vi "Three_Tote.vi"(11 "3_Tote_Enable":bool=TRUE) -> ()   [LabVIEW 2014]
uses:
  General_VI/Global Var.vi
panel:
  in  "Time _To_Drive_1_Tote":i32=8000
  in  "Extend_Flipper_Time":i32=500
  in  "Open_Infeed_time":i32=800
  # "Static Tunning Values"
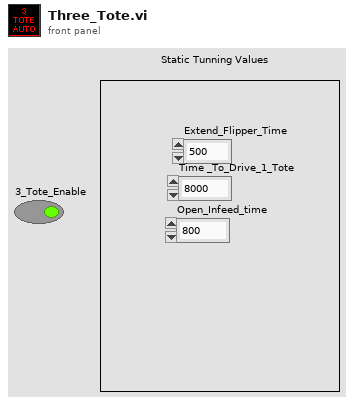
[diagram p1: front panel]
types:
  T1 = cluster{"Open_Infeed_time":i32, "Extend_Flipper_Time":i32, "Time _To_Drive_1_Tote":i32}
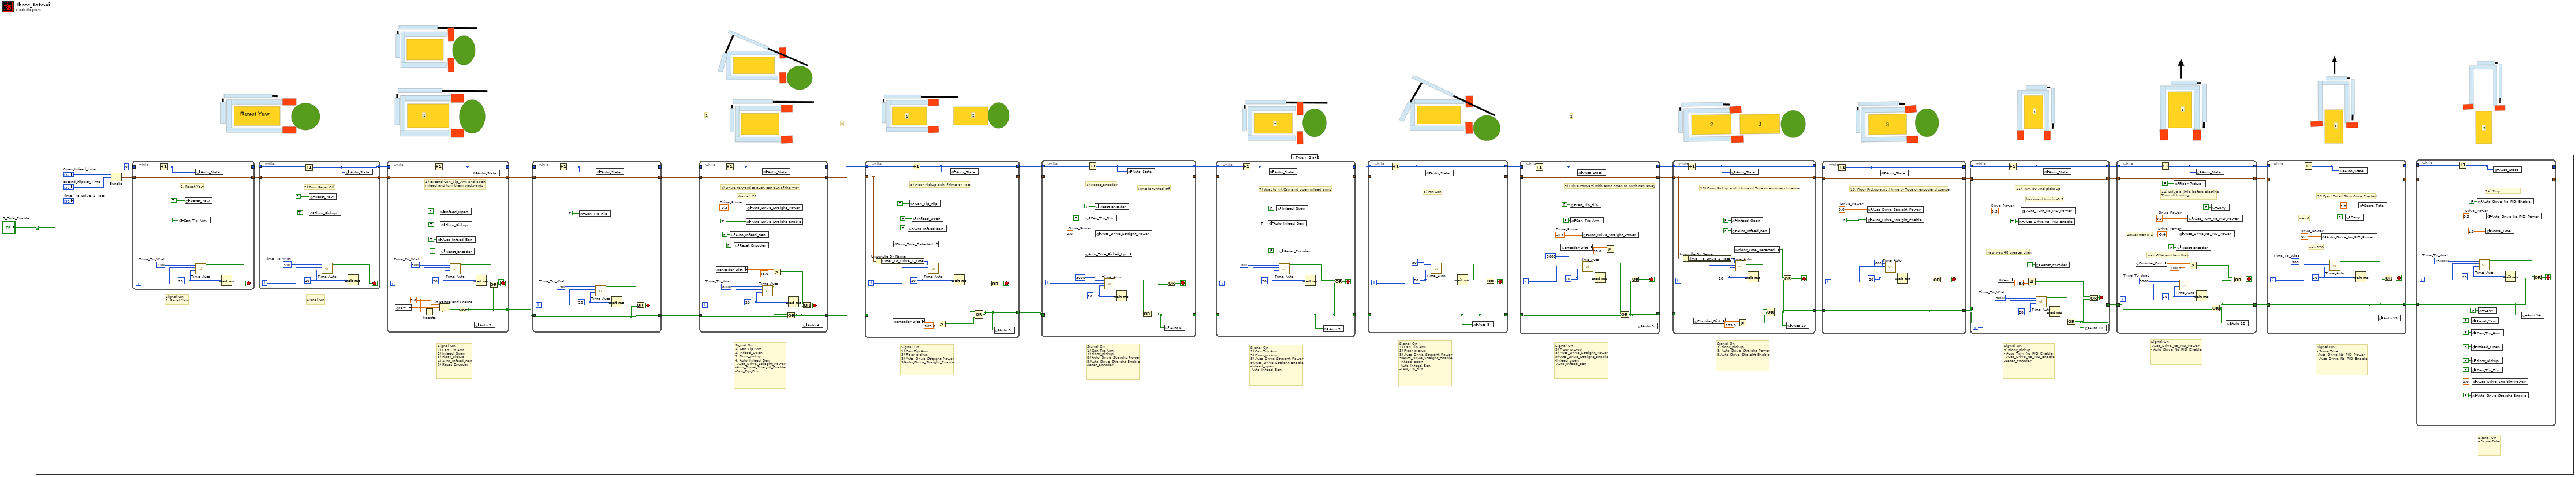
[diagram p0: block diagram]
diagram:
  # "3"
  # "3"
  # "3"
  # "3"
  # "2"
  # "2"
  # "2"
  # "1"
  # "1"
  # "1"
  # "1"
  n1 = case shown="True" "3_Tote_Enable" {
    frame False {
    }
    frame True {
      # "Signal On\n1) Can Tip Arm\n2) Infeed_Open\n3) Floor_pickup\n4) Auto_Infeed_Ben\n- Auto_Drive_Striaght_Power\n-Auto_Drive_Straight_Enable\n-Can_Tip_FLip"
      # "Signal On\n- Score Tote"
      # "Signal On\n- Score Tote\n-Auto_Drive_No_PID_Power\n- Auto_Drive_No_PID_Enable"
      # "Signal On\n-Auto_Drive_No_PID_Power\n- Auto_Drive_No_PID_Enable"
      # "Signal On\n3) Floor_pickup\n- Auto_Turn_No_PID_Enable\n- Auto_Drive_No_PID_Enable\n-Reset_Encoder"
      # "Signal On\n3) Floor_pickup\n8) Auto_Drive_Straight_Power\n9)Auto_Drive_Straight_Enable"
      # "Signal On\n3) Floor_pickup\n8) Auto_Drive_Straight_Power\n9)Auto_Drive_Straight_Enable\n-Infeed_open\n-Auto_Infeed_Ben"
      # "Signal On\n1) Can Tip Arm\n3) Floor_pickup\n8) Auto_Drive_Straight_Power\n9)Auto_Drive_Straight_Enable\n-Infeed_open\n-Auto_Infeed_Ben\n-CAN_Tip_Flip"
      # "Signal On\n1) Can Tip Arm\n3) Floor_pickup\n8) Auto_Drive_Straight_Power\n9)Auto_Drive_Straight_Enable\n-Infeed_open\n-Auto_Infeed_Ben"
      # "Signal On\n1) Can Tip Arm\n3) Floor_pickup\n8) Auto_Drive_Straight_Power\n9)Auto_Drive_Straight_Enable\n-reset_encoder"
      # "Signal On\n1) Can Tip Arm\n3) Floor_pickup\n8) Auto_Drive_Straight_Power\n9)Auto_Drive_Straight_Enable"
      # "Signal On\n1) Can Tip Arm\n2) Infeed_Open\n3) Floor_pickup\n4) Auto_Infeed_Ben\n5) Reset_Encoder"
      # "Signal On"
      # "Signal On\n1) Reset Yaw"
      n2 = Bundle("Open_Infeed_time"="Open_Infeed_time", "Extend_Flipper_Time"="Extend_Flipper_Time", "Time _To_Drive_1_Tote"="Time _To_Drive_1_Tote") -> (w39:T1)  [unwired: 1 in]
      n3 = while {
        tunnel: 0 -> [w266]
        tunnel: [w265] -> w48
        tunnel: w39 -> [w267]
        tunnel: [w267] -> w38
        i -> [w270]
        stop <- w272 stop-if-true
        w271 = u32 20 ("milliseconds to wait")
        w269 = 100  # Time_To_Wiat
        # "1) Reset Yaw"
        n4 = Increment(x=w266) -> (x+1=w265:i32)
        n5 = global write "Global Var.vi" "Can_Tip_Arm"(TRUE) -> ()
        n6 = global write "Global Var.vi" "Reset_Yaw"(TRUE) -> ()
        n7 = global write "Global Var.vi" "Auto_State"(w265) -> ()
        n8 = call "Time_Auto.vi"("Sample_Time"=w271, "Counter"=w270, "Time_to_wait"=w269) -> ("Boolean"=w272:bool)  [unwired: 8 in]
        n9 = Wait (ms)(milliseconds to wait=w271) -> ()  [unwired: 1 out]
      }
      n10 = while {
        tunnel: w48 -> [w257]
        tunnel: [w256] -> w47
        tunnel: w38 -> [w258]
        tunnel: [w258] -> w37
        i -> [w261]
        stop <- w263 stop-if-true
        w262 = u32 20 ("milliseconds to wait")
        w260 = 300  # Time_To_Wiat
        # "2) Turn Reset Off"
        n11 = Increment(x=w257) -> (x+1=w256:i32)
        n12 = global write "Global Var.vi" "Reset_Yaw"(FALSE) -> ()
        n13 = global write "Global Var.vi" "Floor_Pickup"(TRUE) -> ()
        n14 = call "Time_Auto.vi"("Sample_Time"=w262, "Counter"=w261, "Time_to_wait"=w260) -> ("Boolean"=w263:bool)  [unwired: 8 in]
        n15 = global write "Global Var.vi" "Auto_State"(w256) -> ()
        n16 = Wait (ms)(milliseconds to wait=w262) -> ()  [unwired: 1 out]
      }
      n17 = while {
        tunnel: w47 -> [w250]
        tunnel: [w249] -> w11
        tunnel: w37 -> [w251]
        tunnel: [w251] -> w12
        tunnel: [w238] -> w14
        i -> [w253]
        stop <- w240 stop-if-true
        w244 = 5.0 ("upper limit")
        w254 = u32 20 ("milliseconds to wait")
        w252 = 500  # Time_To_Wiat
        # "3) Extend Can_Tip_Arm and open \ninfeed and turn them backwards"
        n18 = global read "Global Var.vi" "Yaw"() -> (w246:dbl)
        n19 = Negate(x=w244) -> (-x=w245:dbl)
        n20 = Increment(x=w250) -> (x+1=w249:i32)
        n21 = global write "Global Var.vi" "Auto_Infeed_Ben"(TRUE) -> ()
        n22 = In Range and Coerce(upper limit=w244, x=w246, lower limit=w245) -> (In Range?=w243:bool)  [unwired: 1 out]
        n23 = global write "Global Var.vi" "Infeed_Open"(FALSE) -> ()
        n24 = global write "Global Var.vi" "Floor_Pickup"(TRUE) -> ()
        n25 = global write "Global Var.vi" "Reset_Encoder"(TRUE) -> ()
        n26 = call "Time_Auto.vi"("Sample_Time"=w254, "Counter"=w253, "Time_to_wait"=w252) -> ("Boolean"=w239:bool)  [unwired: 8 in]
        n27 = Not(x=w243) -> (.not. x?=w238:bool)
        n28 = global write "Global Var.vi" "Auto_State"(w249) -> ()
        n29 = global write "Global Var.vi" "Auto 3"(w238) -> ()
        n30 = Wait (ms)(milliseconds to wait=w254) -> ()  [unwired: 1 out]
        n31 = Or(x=w239, y=w238) -> (x .or. y?=w240:bool)
      }
      n32 = while {
        tunnel: w11 -> [w66]
        tunnel: [w65] -> w10
        tunnel: w12 -> [w67]
        tunnel: [w67] -> w9
        tunnel: w14 -> [w61]
        tunnel: [w61] -> w13
        i -> [w69]
        stop <- w64 stop-if-true
        w70 = u32 20 ("milliseconds to wait")
        w68 = 750  # Time_To_Wiat
        n33 = Increment(x=w66) -> (x+1=w65:i32)
        n34 = global write "Global Var.vi" "Can_Tip_Flip"(TRUE) -> ()
        n35 = call "Time_Auto.vi"("Sample_Time"=w70, "Counter"=w69, "Time_to_wait"=w68) -> ("Boolean"=w62:bool)  [unwired: 8 in]
        n36 = global write "Global Var.vi" "Auto_State"(w65) -> ()
        n37 = Wait (ms)(milliseconds to wait=w70) -> ()  [unwired: 1 out]
        n38 = Or(x=w62, y=w61) -> (x .or. y?=w64:bool)
      }
      n39 = while {
        tunnel: w10 -> [w233]
        tunnel: [w232] -> w33
        tunnel: w9 -> [w234]
        tunnel: [w234] -> w32
        tunnel: w13 -> [w225]
        tunnel: [w222] -> w31
        i -> [w236]
        stop <- w224 stop-if-true
        w231 = -0.3  # Drive_Power
        w237 = u32 20 ("milliseconds to wait")
        w235 = 8000  # Time_To_Wiat
        # "Was at .22"
        # "4) Drive Forward to push can out of the way"
        n40 = global read "Global Var.vi" "Encoder_Dist"() -> (w228:dbl)
        n41 = Increment(x=w233) -> (x+1=w232:i32)
        n42 = global write "Global Var.vi" "Auto_Infeed_Ben"(FALSE) -> ()
        n43 = global write "Global Var.vi" "Reset_Encoder"(FALSE ("Reset_Encoder")) -> ()
        n44 = global write "Global Var.vi" "Auto_Drive_Straight_Enable"(TRUE) -> ()
        n45 = global write "Global Var.vi" "Auto_Drive_Straight_Power"(w231) -> ()
        n46 = call "Time_Auto.vi"("Sample_Time"=w237, "Counter"=w236, "Time_to_wait"=w235) -> ("Boolean"=w226:bool)  [unwired: 8 in]
        n47 = global write "Global Var.vi" "Auto_State"(w232) -> ()
        n48 = Greater?(x=w228, y=43.0) -> (0:w223:bool)
        n49 = Or(x=w226, y=w225) -> (x .or. y?=w222:bool)
        n50 = Wait (ms)(milliseconds to wait=w237) -> ()  [unwired: 1 out]
        n51 = Or(x=w223, y=w222) -> (x .or. y?=w224:bool)
        n52 = global write "Global Var.vi" "Auto 4"(w222) -> ()
      }
      n53 = while {
        tunnel: w33 -> [w218]
        tunnel: [w217] -> w30
        tunnel: w32 -> [w216]
        tunnel: [w216] -> w29
        tunnel: w31 -> [w214]
        tunnel: [w204] -> w2
        i -> [w219]
        stop <- w210 stop-if-true
        w220 = u32 20 ("milliseconds to wait")
        # "5) Floor Pickup exit if time or Tote"
        n54 = Unbundle By Name(w216) -> ("Time _To_Drive_1_Tote"=w215:i32)
        n55 = global read "Global Var.vi" "Encoder_Dist"() -> (w208:dbl)
        n56 = global read "Global Var.vi" "Floor_Tote_Detected"() -> (w209:bool)
        n57 = global write "Global Var.vi" "Auto_Infeed_Ben"(FALSE) -> ()
        n58 = global write "Global Var.vi" "Can_Tip_Flip"(FALSE) -> ()
        n59 = Increment(x=w218) -> (x+1=w217:i32)
        n60 = global write "Global Var.vi" "Infeed_Open"(FALSE) -> ()
        n61 = call "Time_Auto.vi"("Sample_Time"=w220, "Counter"=w219, "Time_to_wait"=w215) -> ("Boolean"=w213:bool)  [unwired: 8 in]
        n62 = Greater?(x=w208, y=105.0) -> (0:w207:bool)
        n63 = global write "Global Var.vi" "Auto_State"(w217) -> ()
        n64 = Wait (ms)(milliseconds to wait=w220) -> ()  [unwired: 1 out]
        n65 = Compound Arithmetic op=OR(w213, w214, w207) -> (w204:bool)
        n66 = Or(x=w209, y=w204) -> (x .or. y?=w210:bool)
        n67 = global write "Global Var.vi" "Auto 5"(w204) -> ()
      }
      n68 = while {
        tunnel: w30 -> [w98]
        tunnel: [w97] -> w15
        tunnel: w29 -> [w96]
        tunnel: [w96] -> w22
        tunnel: w2 -> [_]
        tunnel: [w88] -> w28
        tunnel: w2 -> [w89]
        i -> [w99]
        stop <- w95 stop-if-true
        w91 = 0.0  # Drive_Power
        w100 = u32 20 ("milliseconds to wait")
        # "TIme is turned off"
        # "6) Reset_Encoder"
        n69 = global read "Global Var.vi" "Auto_Tote_Picked_Up"() -> (w92:bool)
        n70 = global write "Global Var.vi" "Can_Tip_Flip"(TRUE) -> ()
        n71 = Increment(x=w98) -> (x+1=w97:i32)
        n72 = global write "Global Var.vi" "Reset_Encoder"(TRUE) -> ()
        n73 = global write "Global Var.vi" "Auto_Drive_Straight_Power"(w91) -> ()
        n74 = call "Time_Auto.vi"("Sample_Time"=w100, "Counter"=w99, "Time_to_wait"=3000) -> ("Boolean"=w90:bool)  [unwired: 8 in]
        n75 = Wait (ms)(milliseconds to wait=w100) -> ()  [unwired: 1 out]
        n76 = global write "Global Var.vi" "Auto_State"(w97) -> ()
        n77 = Compound Arithmetic op=OR(w90, w89) -> (w88:bool)
        n78 = global write "Global Var.vi" "Auto 6"(w88) -> ()
        n79 = Or(x=w92, y=w88) -> (x .or. y?=w95:bool)
      }
      n80 = while {
        tunnel: [w201] -> w46
        tunnel: w28 -> [w192]
        tunnel: [w192] -> w27
        tunnel: w22 -> [w194]
        tunnel: [w194] -> w21
        tunnel: w15 -> [w193]
        i -> [w202]
        stop <- w199 stop-if-true
        w203 = u32 20 ("milliseconds to wait")
        # "7) Wiat to hit Can and open infeed arms"
        n81 = Increment(x=w193) -> (x+1=w201:i32)
        n82 = global write "Global Var.vi" "Auto_Infeed_Ben"(TRUE) -> ()
        n83 = global write "Global Var.vi" "Auto_State"(w201) -> ()
        n84 = global write "Global Var.vi" "Infeed_Open"(FALSE ("Infeed_Open")) -> ()
        n85 = global write "Global Var.vi" "Reset_Encoder"(FALSE) -> ()
        n86 = call "Time_Auto.vi"("Sample_Time"=w203, "Counter"=w202, "Time_to_wait"=100) -> ("Boolean"=w198:bool)  [unwired: 8 in]
        n87 = Wait (ms)(milliseconds to wait=w203) -> ()  [unwired: 1 out]
        n88 = global write "Global Var.vi" "Auto 7"(w192) -> ()
        n89 = Or(x=w198, y=w192) -> (x .or. y?=w199:bool)
      }
      n90 = while {
        tunnel: w46 -> [w189]
        tunnel: [w188] -> w26
        tunnel: w27 -> [w183]
        tunnel: [w183] -> w24
        tunnel: w21 -> [w185]
        tunnel: [w185] -> w20
        i -> [w190]
        stop <- w187 stop-if-true
        w191 = u32 20 ("milliseconds to wait")
        # "8) HIt Can"
        n91 = Increment(x=w189) -> (x+1=w188:i32)
        n92 = global write "Global Var.vi" "Auto_State"(w188) -> ()
        n93 = call "Time_Auto.vi"("Sample_Time"=w191, "Counter"=w190, "Time_to_wait"=50) -> ("Boolean"=w186:bool)  [unwired: 8 in]
        n94 = Wait (ms)(milliseconds to wait=w191) -> ()  [unwired: 1 out]
        n95 = global write "Global Var.vi" "Auto 8"(w183) -> ()
        n96 = Or(x=w186, y=w183) -> (x .or. y?=w187:bool)
      }
      n97 = while {
        tunnel: [w83] -> w25
        tunnel: w26 -> [w82]
        tunnel: w24 -> [w79]
        tunnel: [w72] -> w23
        tunnel: [w74] -> _
        tunnel: w20 -> [w74]
        tunnel: [w74] -> w19
        i -> [w85]
        stop <- w84 stop-if-true
        w71 = -0.3  # Drive_Power
        w86 = u32 20 ("milliseconds to wait")
        # "9) Drive Forward with arms open to push can away"
        n98 = Increment(x=w82) -> (x+1=w83:i32)
        n99 = global read "Global Var.vi" "Encoder_Dist"() -> (w78:dbl)
        n100 = global write "Global Var.vi" "Can_Tip_Flip"(FALSE ("Infeed_Open")) -> ()
        n101 = global write "Global Var.vi" "Can_Tip_Arm"(FALSE ("Infeed_Open")) -> ()
        n102 = global write "Global Var.vi" "Auto_State"(w83) -> ()
        n103 = global write "Global Var.vi" "Auto_Drive_Straight_Power"(w71) -> ()
        n104 = call "Time_Auto.vi"("Sample_Time"=w86, "Counter"=w85, "Time_to_wait"=3000) -> ("Boolean"=w81:bool)  [unwired: 8 in]
        n105 = Wait (ms)(milliseconds to wait=w86) -> ()  [unwired: 1 out]
        n106 = Greater?(x=w78, y=30.0) -> (0:w76:bool)
        n107 = Compound Arithmetic op=OR(w81, w79) -> (w72:bool)
        n108 = Or(x=w76, y=w72) -> (x .or. y?=w84:bool)
        n109 = global write "Global Var.vi" "Auto 9"(w72) -> ()
      }
      n110 = while {
        tunnel: [w178] -> w8
        tunnel: [w167] -> w5
        tunnel: w25 -> [w175]
        tunnel: w23 -> [w172]
        tunnel: w19 -> [w170]
        tunnel: [w170] -> w3
        i -> [w181]
        stop <- w180 stop-if-true
        w182 = u32 20 ("milliseconds to wait")
        # "10) Floor Pickup exit if time or Tote or encoder distance"
        n111 = Unbundle By Name(w170) -> ("Time _To_Drive_1_Tote"=w177:i32)
        n112 = Increment(x=w175) -> (x+1=w178:i32)
        n113 = global read "Global Var.vi" "Encoder_Dist"() -> (w173:dbl)
        n114 = global write "Global Var.vi" "Auto_State"(w178) -> ()
        n115 = global write "Global Var.vi" "Infeed_Open"(FALSE ("Infeed_Open")) -> ()
        n116 = global write "Global Var.vi" "Auto_Infeed_Ben"(FALSE) -> ()
        n117 = global read "Global Var.vi" "Floor_Tote_Detected"() -> (w179:bool)
        n118 = call "Time_Auto.vi"("Sample_Time"=w182, "Counter"=w181, "Time_to_wait"=w177) -> ("Boolean"=w176:bool)  [unwired: 8 in]
        n119 = Greater?(x=w173, y=105.0) -> (0:w171:bool)
        n120 = Wait (ms)(milliseconds to wait=w182) -> ()  [unwired: 1 out]
        n121 = Compound Arithmetic op=OR(w176, w172, w171) -> (w167:bool)
        n122 = Or(x=w179, y=w167) -> (x .or. y?=w180:bool)
        n123 = global write "Global Var.vi" "Auto 10"(w167) -> ()
      }
      n124 = while {
        tunnel: [w58] -> w7
        tunnel: w8 -> [w57]
        tunnel: w3 -> [w56]
        tunnel: [w56] -> w6
        tunnel: w5 -> [w53]
        tunnel: [w53] -> w4
        i -> [w59]
        stop <- w55 stop-if-true
        w51 = 0.0  # Drive_Power
        w60 = u32 20 ("milliseconds to wait")
        # "10) Floor Pickup exit if time or Tote or encoder distance"
        n125 = Increment(x=w57) -> (x+1=w58:i32)
        n126 = global write "Global Var.vi" "Auto_Drive_Straight_Enable"(FALSE) -> ()
        n127 = global write "Global Var.vi" "Auto_Drive_Straight_Power"(w51) -> ()
        n128 = global write "Global Var.vi" "Auto_State"(w58) -> ()
        n129 = call "Time_Auto.vi"("Sample_Time"=w60, "Counter"=w59, "Time_to_wait"=800) -> ("Boolean"=w54:bool)  [unwired: 8 in]
        n130 = Wait (ms)(milliseconds to wait=w60) -> ()  [unwired: 1 out]
        n131 = Or(x=w54, y=w53) -> (x .or. y?=w55:bool)
      }
      n132 = while {
        tunnel: w7 -> [w166]
        tunnel: [w165] -> w45
        tunnel: w4 -> [w157]
        tunnel: [w154] -> w36
        tunnel: w6 -> [w162]
        tunnel: [w162] -> w18
        i -> [w158]
        stop <- w155 stop-if-true
        w160 = u32 20 ("milliseconds to wait")
        w159 = 3000  # Time_To_Wiat
        w164 = 0.5  # Drive_Power
        # "yaw was 48 greater than"
        # "backward turn is -0.5"
        # "11) Turn 90 And picks up"
        n133 = global read "Global Var.vi" "Yaw"() -> (w153:dbl)
        n134 = Increment(x=w166) -> (x+1=w165:i32)
        n135 = global write "Global Var.vi" "Auto_Drive_No_PID_Enable"(TRUE ("Auto_Drive_No_PID_Enable")) -> ()
        n136 = global write "Global Var.vi" "Auto_Turn_No_PID_Power"(w164) -> ()
        n137 = Less Or Equal?(x=w153, y=-48.0) -> (x <= y?=w151:bool)
        n138 = global write "Global Var.vi" "Reset_Encoder"(TRUE ("Reset_Encoder")) -> ()
        n139 = call "Time_Auto.vi"("Sample_Time"=w160, "Counter"=w158, "Time_to_wait"=w159) -> ("Boolean"=w156:bool)  [unwired: 8 in]
        n140 = global write "Global Var.vi" "Auto_State"(w165) -> ()
        n141 = Wait (ms)(milliseconds to wait=w160) -> ()  [unwired: 1 out]
        n142 = Compound Arithmetic op=OR(w156, w157) -> (w154:bool)
        n143 = global write "Global Var.vi" "Auto 11"(w154) -> ()
        n144 = Or(x=w151, y=w154) -> (x .or. y?=w155:bool)
      }
      n145 = while {
        tunnel: w45 -> [w146]
        tunnel: [w145] -> w44
        tunnel: w36 -> [w140]
        tunnel: [w137] -> w35
        tunnel: w18 -> [w143]
        tunnel: [w143] -> w17
        i -> [w149]
        stop <- w138 stop-if-true
        w144 = 0.0  # Drive_Power
        w147 = -0.4  # Drive_Power
        w150 = u32 20 ("milliseconds to wait")
        w148 = 5000  # Time_To_Wiat
        # "was -114 and less than"
        # "Power was 0.4"
        # "12) Drive a little before ejecting\nTurn off turning"
        n146 = global read "Global Var.vi" "Encoder_Dist"() -> (w136:dbl)
        n147 = Increment(x=w146) -> (x+1=w145:i32)
        n148 = global write "Global Var.vi" "Floor_Pickup"(FALSE) -> ()
        n149 = global write "Global Var.vi" "Reset_Encoder"(FALSE ("Reset_Encoder")) -> ()
        n150 = global write "Global Var.vi" "Auto_Drive_No_PID_Power"(w147) -> ()
        n151 = call "Time_Auto.vi"("Sample_Time"=w150, "Counter"=w149, "Time_to_wait"=w148) -> ("Boolean"=w141:bool)  [unwired: 8 in]
        n152 = global write "Global Var.vi" "Auto_Turn_No_PID_Power"(w144) -> ()
        n153 = Greater?(x=w136, y=100.0) -> (0:w134:bool)
        n154 = global write "Global Var.vi" "Auto_State"(w145) -> ()
        n155 = Wait (ms)(milliseconds to wait=w150) -> ()  [unwired: 1 out]
        n156 = global write "Global Var.vi" "Carry"(TRUE ("Carry")) -> ()
        n157 = Compound Arithmetic op=OR(w141, w140) -> (w137:bool)
        n158 = global write "Global Var.vi" "Auto 12"(w137) -> ()
        n159 = Or(x=w134, y=w137) -> (x .or. y?=w138:bool)
      }
      n160 = while {
        tunnel: w44 -> [w128]
        tunnel: [w127] -> w43
        tunnel: w35 -> [w122]
        tunnel: [w122] -> w34
        tunnel: w17 -> [w125]
        tunnel: [w125] -> w16
        i -> [w131]
        stop <- w124 stop-if-true
        w126 = 0.4  # Drive_Power
        w132 = u32 20 ("milliseconds to wait")
        w130 = 500  # Time_To_Wiat
        # "was 120"
        # "was 0"
        # "13)Eject Totes Stop Once Ejected"
        n161 = Increment(x=w128) -> (x+1=w127:i32)
        n162 = global write "Global Var.vi" "Auto_Drive_No_PID_Power"(w126) -> ()
        n163 = call "Time_Auto.vi"("Sample_Time"=w132, "Counter"=w131, "Time_to_wait"=w130) -> ("Boolean"=w123:bool)  [unwired: 8 in]
        n164 = global write "Global Var.vi" "Auto_State"(w127) -> ()
        n165 = global write "Global Var.vi" "Carry"(FALSE ("Carry")) -> ()
        n166 = Wait (ms)(milliseconds to wait=w132) -> ()  [unwired: 1 out]
        n167 = global write "Global Var.vi" "Score_Tote"(1.0) -> ()
        n168 = global write "Global Var.vi" "Auto 13"(w122) -> ()
        n169 = Or(x=w123, y=w122) -> (x .or. y?=w124:bool)
      }
      n170 = while {
        tunnel: w43 -> [w116]
        tunnel: [w115] -> _
        tunnel: w34 -> [w102]
        tunnel: w16 -> [w105]
        tunnel: [w105] -> _
        i -> [w119]
        stop <- w104 stop-if-true
        w113 = 0.0  # Drive_Power
        w120 = u32 20 ("milliseconds to wait")
        w118 = 150000  # Time_To_Wiat
        # "14) Stop"
        n171 = Increment(x=w116) -> (x+1=w115:i32)
        n172 = global write "Global Var.vi" "Reset_Yaw"(FALSE ("Reset_Yaw")) -> ()
        n173 = global write "Global Var.vi" "Can_Tip_Arm"(FALSE ("Can_Tip_Arm")) -> ()
        n174 = global write "Global Var.vi" "Infeed_Open"(FALSE ("Infeed_Open")) -> ()
        n175 = global write "Global Var.vi" "Floor_Pickup"(FALSE ("Floor_Pickup")) -> ()
        n176 = global write "Global Var.vi" "Can_Tip_Flip"(FALSE ("Can_Tip_Flip")) -> ()
        n177 = global write "Global Var.vi" "Auto_Drive_Straight_Enable"(FALSE ("Auto_Drive_Straight_Enable")) -> ()
        n178 = global write "Global Var.vi" "Auto_Drive_Straight_Power"(0.0 ("Auto_Drive_Straight_Power")) -> ()
        n179 = global write "Global Var.vi" "Auto_Drive_No_PID_Enable"(FALSE ("Auto_Drive_No_PID_Enable")) -> ()
        n180 = global write "Global Var.vi" "Carry"(FALSE ("Carry")) -> ()
        n181 = call "Time_Auto.vi"("Sample_Time"=w120, "Counter"=w119, "Time_to_wait"=w118) -> ("Boolean"=w103:bool)  [unwired: 8 in]
        n182 = global write "Global Var.vi" "Score_Tote"(1.0) -> ()
        n183 = global write "Global Var.vi" "Auto_Drive_No_PID_Power"(w113) -> ()
        n184 = global write "Global Var.vi" "Auto_State"(w115) -> ()
        n185 = Wait (ms)(milliseconds to wait=w120) -> ()  [unwired: 1 out]
        n186 = global write "Global Var.vi" "Auto 14"(w102) -> ()
        n187 = Or(x=w103, y=w102) -> (x .or. y?=w104:bool)
      }
    }
  }
